vi "Read Path.vi"(8 "error in (no error)":errorcluster, 11 "Database Manager in":refnum<class "Database Manager.lvclass">) -> (0 "error out":errorcluster, 2 "Path":path, 3 "Database Manager out":refnum<class "Database Manager.lvclass">)   [LabVIEW 2021, in "Database Manager.lvclass"]
uses:
  Database Manager.lvclass
  Database Manager.lvclass/Database Manager.ctl
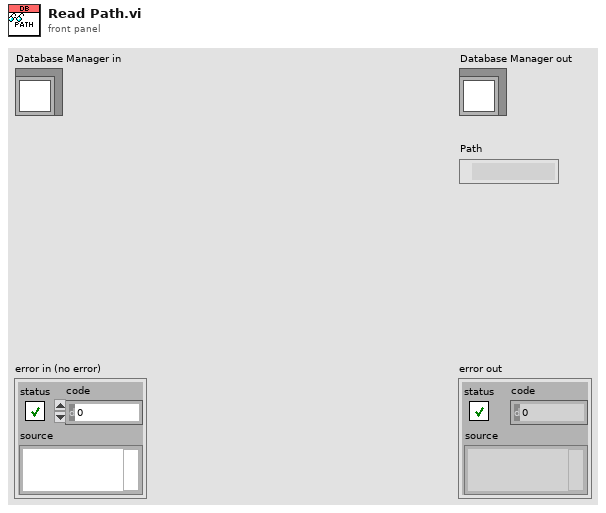
[diagram p1: front panel]
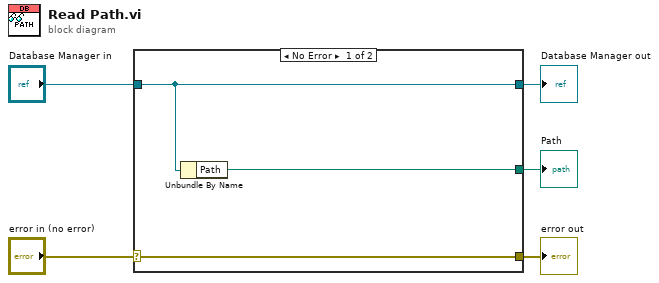
[diagram p0: block diagram]
diagram:
  n1 = case shown="No Error" "error in (no error)" {
    selector: "error in (no error)" -> [w8 w9]
    tunnel: [w8 w9] -> w4
    tunnel: [w7 w10] -> w2
    tunnel: "Database Manager in" -> [w7 w10]
    tunnel: [w6 _] -> w1
    frame No Error {
      n2 = Unbundle By Name(w7) -> ("Path"=w6:path)
    }
    frame Error {
    }
  }
  "error out" <- w4
  "Database Manager out" <- w2
  "Path" <- w1
